vi "Page_Advanced_Initialize.vi"(6 "ctl references":T1, 8 "error in (no error)":errorcluster, 11 "AB_PackedLibrary in":refnum<class "AB_PackedLibrary.lvclass">) -> (0 "error out":errorcluster, 3 "AB_PackedLibrary out":refnum<class "AB_PackedLibrary.lvclass">)   [LabVIEW 2020, in "AB_PackedLibrary.lvclass"]
uses:
  <vilib>/AppBuilder/AB_Classes/PackedLib/AB_PackedLibrary.lvclass
  <resource>/Framework/Providers/Builds/AppBuilder/AB_UI_Page_Advanced_References.ctl
  <resource>/Framework/Providers/Common/provcom_StringGlobals.vi
  <vilib>/AppBuilder/AB_Classes/TargetFile/AB_Targetfile.lvclass
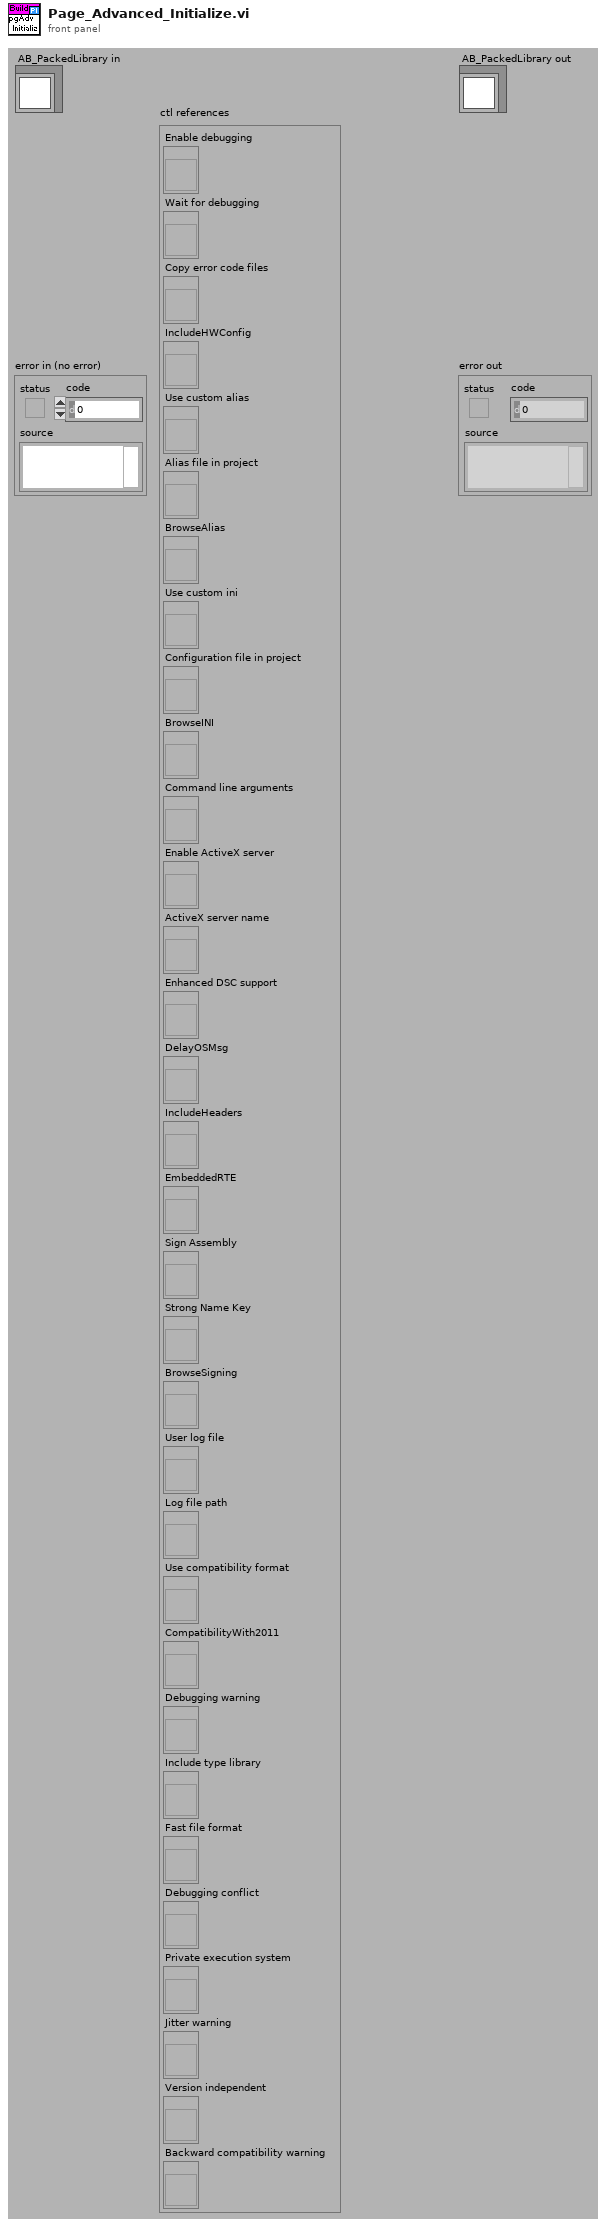
[diagram p1: front panel]
types:
  T1 = typedef "AB_UI_Page_Advanced_References.ctl" = cluster{"Enable debugging":refnum<vi>, "Wait for debugging":refnum<vi>, "Copy error code files":refnum<vi>, "IncludeHWConfig":refnum<vi>, "Use custom alias":refnum<vi>, "Alias file in project":refnum<vi>, "BrowseAlias":refnum<vi>, "Use custom ini":refnum<vi>, "Configuration file in project":refnum<vi>, "BrowseINI":refnum<vi>, "Command line arguments":refnum<vi>, "Enable ActiveX server":refnum<vi>, "ActiveX server name":refnum<vi>, "Enhanced DSC support":refnum<vi>, "DelayOSMsg":refnum<vi>, "IncludeHeaders":refnum<vi>, "EmbeddedRTE":refnum<vi>, "Sign Assembly":refnum<vi>, "Strong Name Key":refnum<vi>, "BrowseSigning":refnum<vi>, "User log file":refnum<vi>, "Log file path":refnum<vi>, "Use compatibility format":refnum<vi>, "CompatibilityWith2011":refnum<vi>, "Debugging warning":refnum<vi>, "Include type library":refnum<vi>, "Fast file format":refnum<vi>, "Debugging conflict":refnum<vi>, "Private execution system":refnum<vi>, "Jitter warning":refnum<vi>, "Version independent":refnum<vi>, "Backward compatibility warning":refnum<vi>}
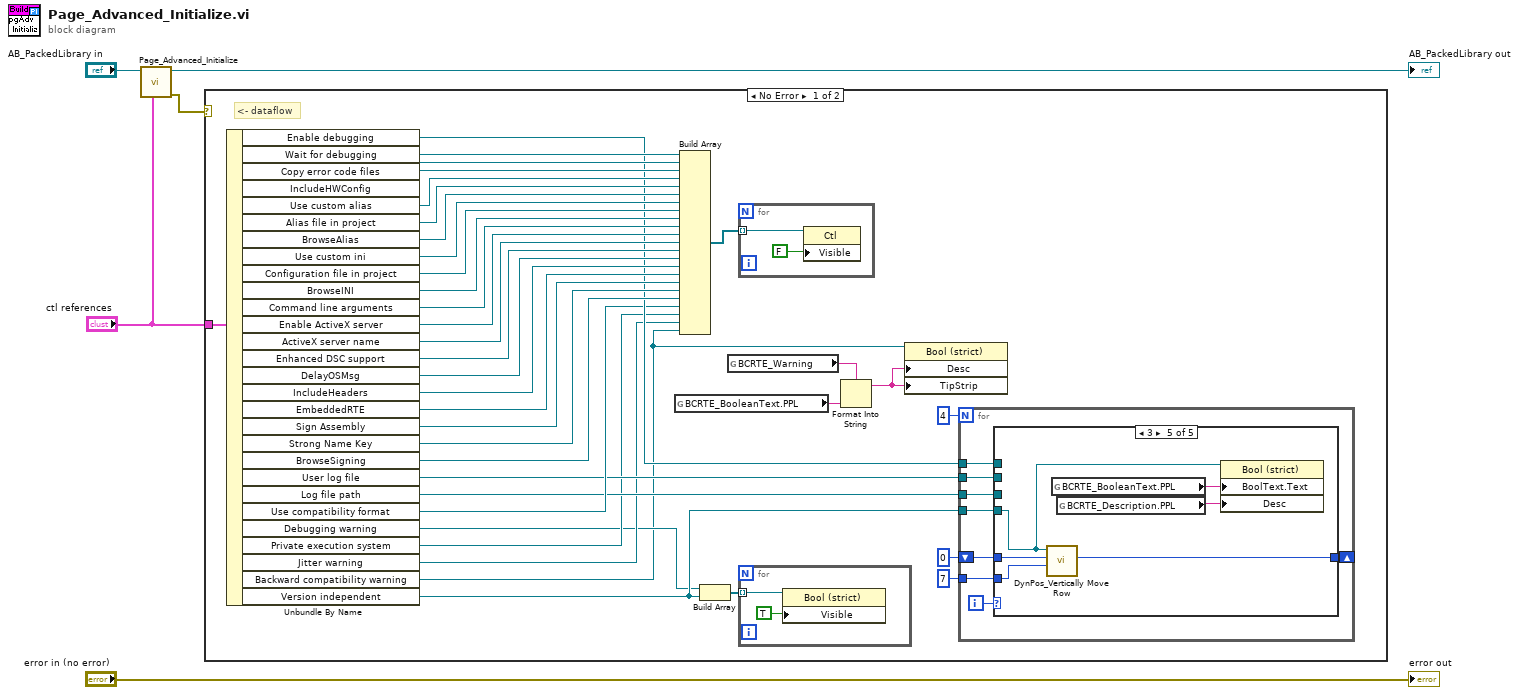
[diagram p0: block diagram]
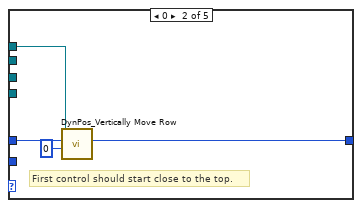
[diagram p3: hidden frame]
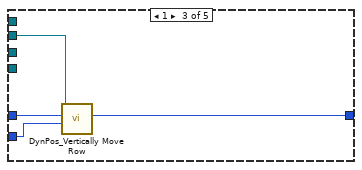
[diagram p4: hidden frame]
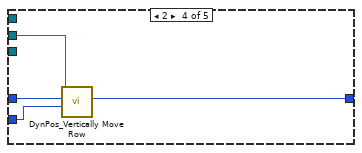
[diagram p5: hidden frame]
diagram:
  n1 = call-parent "Page_Advanced_Initialize.vi"("ctl references"="ctl references", "AB_Build in"="AB_PackedLibrary in") -> ("error out"=w3:errorcluster, "AB_Build out"=→"AB_PackedLibrary out":refnum<class "AB_PackedLibrary.lvclass">)  [unwired: 1 in, 7 out]
  n2 = case shown="No Error" w3 {
    tunnel: "ctl references" -> [w42 _]
    frame No Error {
      # "<- dataflow"
      n3 = Unbundle By Name(w42) -> ("Enable debugging"=w18:refnum<vi>, "Wait for debugging"=w41:refnum<vi>, "Copy error code files"=w40:refnum<vi>, "IncludeHWConfig"=w39:refnum<vi>, "Use custom alias"=w38:refnum<vi>, "Alias file in project"=w37:refnum<vi>, "BrowseAlias"=w36:refnum<vi>, "Use custom ini"=w35:refnum<vi>, "Configuration file in project"=w34:refnum<vi>, "BrowseINI"=w33:refnum<vi>, "Command line arguments"=w32:refnum<vi>, "Enable ActiveX server"=w31:refnum<vi>, "ActiveX server name"=w30:refnum<vi>, "Enhanced DSC support"=w29:refnum<vi>, "DelayOSMsg"=w27:refnum<vi>, "IncludeHeaders"=w26:refnum<vi>, "EmbeddedRTE"=w25:refnum<vi>, "Sign Assembly"=w24:refnum<vi>, "Strong Name Key"=w23:refnum<vi>, "BrowseSigning"=w22:refnum<vi>, "User log file"=w16:refnum<vi>, "Log file path"=w15:refnum<vi>, "Use compatibility format"=w17:refnum<vi>, "Debugging warning"=w10:refnum<vi>, "Private execution system"=w14:refnum<vi>, "Jitter warning"=w13:refnum<vi>, "Backward compatibility warning"=w6:refnum<vi>, "Version independent"=w11:refnum<vi>)
      n4 = global read "provcom_StringGlobals.vi" "BCRTE_BooleanText.PPL"() -> (w8:string)
      n5 = Build Array(w41, w40, w39, w38, w37, w36, w35, w34, w33, w32, w31, w30, w29, w27, w26, w25, w24, w23, w22, w17, w14, w13, w6) -> (w28:refnum<vi>[])
      n6 = Build Array(w10, w11) -> (w12:refnum<vi>[])
      n7 = global read "provcom_StringGlobals.vi" "BCRTE_Warning"() -> (w9:string)
      n8 = for {
        tunnel: w28 -> [w73] mode=indexing
        n9 = property class="Ctl"(reference=w73, "Visible"=FALSE) -> ()  [unwired: 1 in, 2 out]
      }
      n10 = for {
        tunnel: w12 -> [w44] mode=indexing
        n11 = property class="Bool (strict)"(reference=w44, "Visible"=TRUE) -> ()  [unwired: 1 in, 2 out]
      }
      n12 = Format Into String(format string=w9, w8) -> (resulting string=w7:string)  [unwired: 2 in, 1 out]
      n13 = property class="Bool (strict)"(reference=w6, "Desc"=w7, "TipStrip"=w7) -> ()  [unwired: 1 in, 2 out]
      n14 = for {
        N: 4 -> [_]
        tunnel: w16 -> [w51]
        tunnel: w15 -> [w50]
        shift-right: [w49] -> _
        shift-left: 0 ("Bottom pixel") -> [w48]
        tunnel: 7 ("Bottom pixel") -> [w47]
        tunnel: w18 -> [w46]
        tunnel: w11 -> [w45]
        i -> [w52]
        n15 = case shown="3" w52 {
          tunnel: w51 -> [_ _ w58 _ _]
          tunnel: w50 -> [_ _ _ w62 _]
          tunnel: [w53 w56 w61 w65 w71] -> w49
          tunnel: w48 -> [w53 w55 w60 w64 w70]
          tunnel: w47 -> [_ _ w59 w63 w69]
          tunnel: w46 -> [_ w54 _ _ _]
          tunnel: w45 -> [_ _ _ _ w68]
          frame Default {
          }
          frame 0 {
            # "First control should start close to the top."
            n16 = call <vilib>:"DynPos_Vertically Move Row.vi"("Pixel separation (6)"=0, "Bottom of last control"=w55, "Control"=w54) -> ("Bottom pixel"=w56:i32)  [unwired: 1 in, 7 out]
          }
          frame 1 {
            n17 = call <vilib>:"DynPos_Vertically Move Row.vi"("Pixel separation (6)"=w59, "Bottom of last control"=w60, "Control"=w58) -> ("Bottom pixel"=w61:i32)  [unwired: 1 in, 7 out]
          }
          frame 2 {
            n18 = call <vilib>:"DynPos_Vertically Move Row.vi"("Pixel separation (6)"=w63, "Bottom of last control"=w64, "Control"=w62) -> ("Bottom pixel"=w65:i32)  [unwired: 1 in, 7 out]
          }
          frame 3 {
            n19 = call <vilib>:"DynPos_Vertically Move Row.vi"("Pixel separation (6)"=w69, "Bottom of last control"=w70, "Control"=w68) -> ("Bottom pixel"=w71:i32)  [unwired: 1 in, 7 out]
            n20 = global read "provcom_StringGlobals.vi" "BCRTE_BooleanText.PPL"() -> (w67:string)
            n21 = global read "provcom_StringGlobals.vi" "BCRTE_Description.PPL"() -> (w66:string)
            n22 = property class="Bool (strict)"(reference=w68, "BoolText.Text"=w67, "Desc"=w66) -> ()  [unwired: 1 in, 2 out]
          }
        }
      }
    }
    frame Error {
    }
  }
  "error out" <- "error in (no error)"
